vi "neo.vi"() -> ()   [LabVIEW 2012]
uses:
  E:/Kinect/Neobotix/CSInterface/RosBridgeDotNet.dll
  RosBridgeDotNet.dll
panel:
  out "container2":dbl[](graph)
  in  "MelyIP":u16(ring) items=["192.168.0.152", "127.0.0.1"]
  out "Graph":dbl[](graph)
  in  "gear":i32(knob)=12 scale=20.0..5.0
  in  "0seb":bool
  in  "Jobb":dbl(slide) scale=-2.0..2.0
  in  "Bal":dbl(slide) scale=-2.0..2.0 scale format="%0#1_1g"
  out "Joy":picture
  in  "Disconn":bool
  out "IPEredmeny":T1(array[cluster]) {"Status" items=["Success"=0, "DestinationNetworkUnreachable"=11002, "DestinationHostUnreachable"=11003, "DestinationProhibited, DestinationProtocolUnreachable"=11004, "DestinationPortUnreachable"=11005, "NoResources"=11006, "BadOption"=11007, "HardwareError"=11008, "PacketTooBig"=11009, "TimedOut"=11010, "BadRoute"=11012, "TtlExpired"=11013, "TtlReassemblyTimeExceeded"=11014, "ParameterProblem"=11015, "SourceQuench"=11016, "BadDestination"=11018, "DestinationUnreachable"=11040, "TimeExceeded"=11041, "BadHeader"=11042, "UnrecognizedNextHeader"=11043, "IcmpError"=11044, "DestinationScopeMismatch"=11045, "Unknown"=-1]}
  in  "Ping":bool
  in  "MessN":bool
  out "Error Out":errorcluster
  in  "Connnect":bool
  out "Connected":bool
  in  "Stop Button":bool
  out "container1":dbl[](graph)
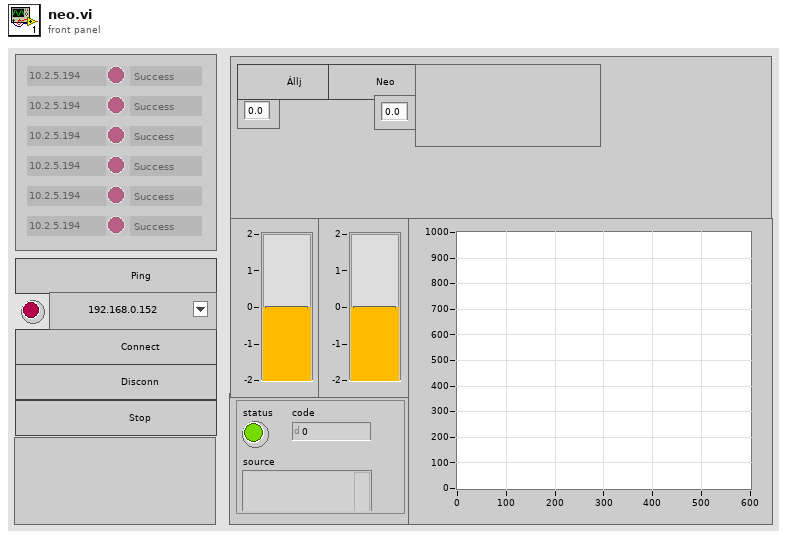
[diagram p1: front panel]
types:
  T1 = cluster{"pingelhet":bool, "IpAddress":string, "Status":i32}[]
  T2 = cluster{"Width":u16, "Style":enum32{"Solid", "Dash", "Dot", "DashDot", "DashDotDot"}}
  T3 = cluster{"left":i16, "top":i16, "right":i16, "bottom":i16}
  T4 = cluster{"pingelhet":bool, "IpAddress":string, "Status":i32}
  T5 = typedef "LVMouseTypeDef.ctl" = cluster{"Mouse Position":cluster{"X":i32, "Y":i32}, "Mouse Modifiers":cluster{"Button Down":bool, "Shift Mod":bool, "Menu Mod":bool, "Option Mod":bool}}
  T6 = typedef "LVBoundsTypeDef.ctl" = cluster{"Width":u32, "Height":u32}
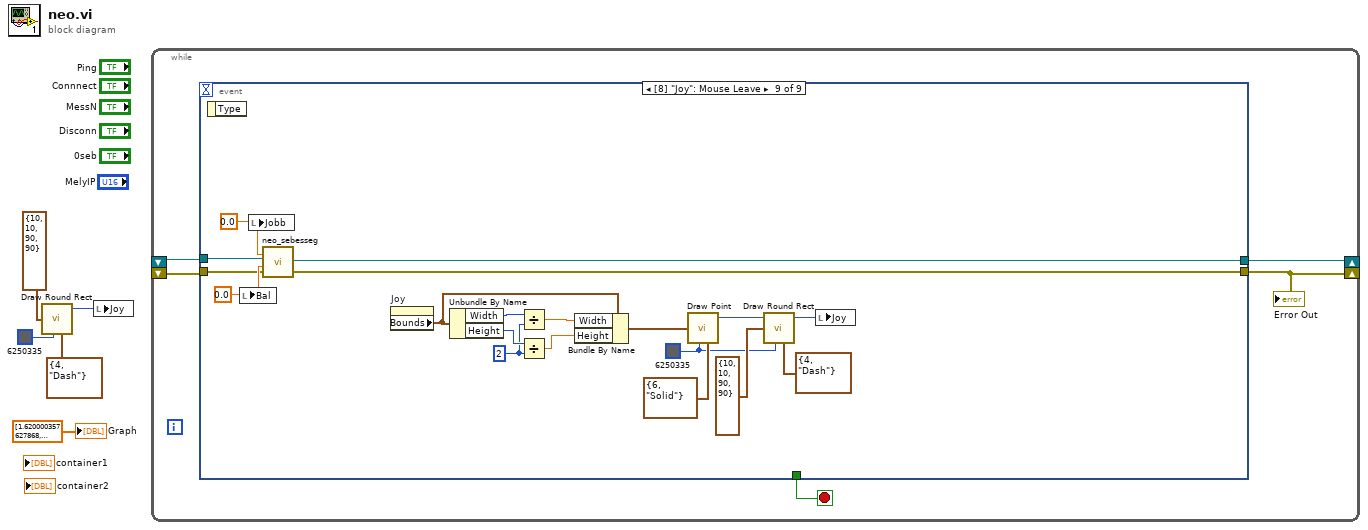
[diagram p0: block diagram]
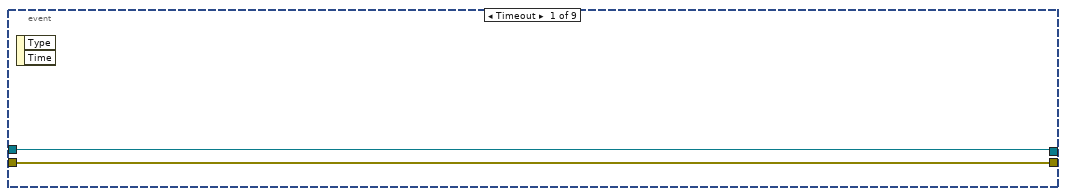
[diagram p2: hidden frame]
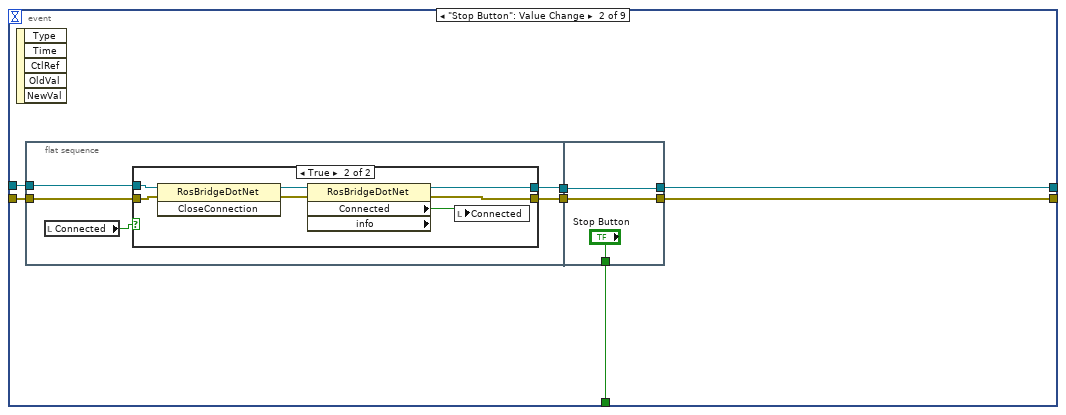
[diagram p3: hidden frame]
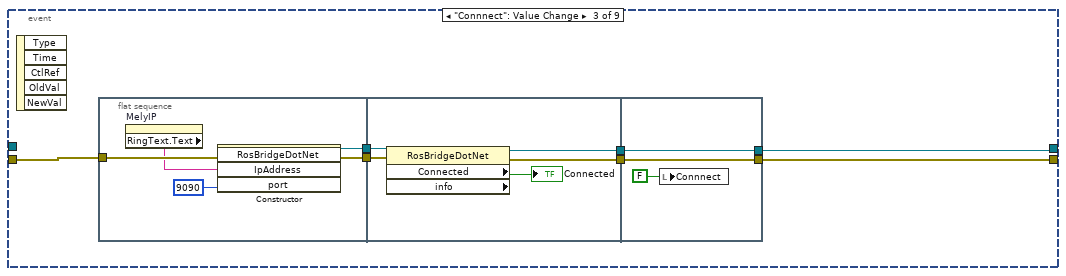
[diagram p5: hidden frame]
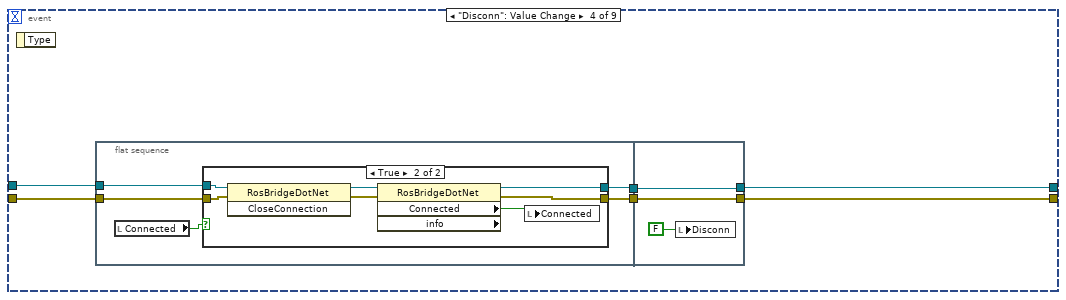
[diagram p6: hidden frame]
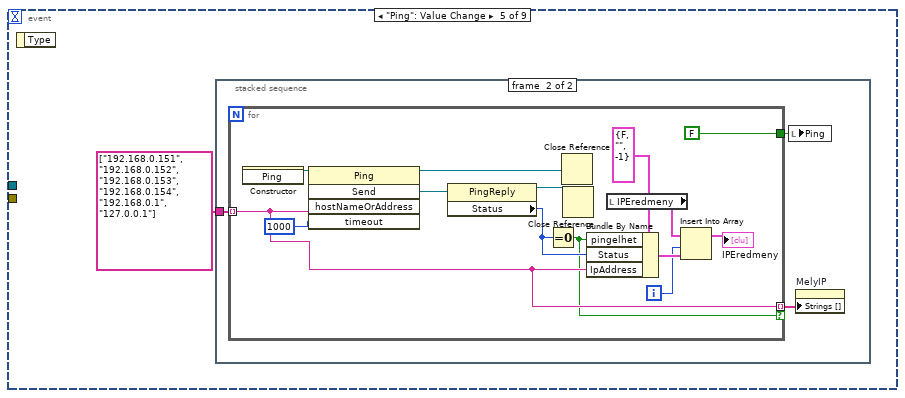
[diagram p8: hidden frame]
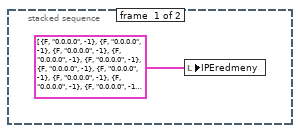
[diagram p9: hidden frame]
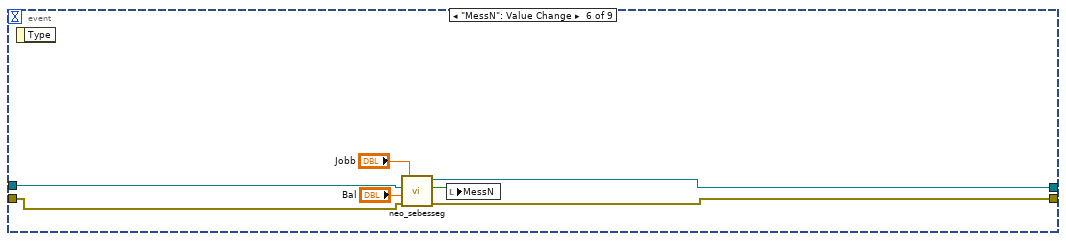
[diagram p10: hidden frame]
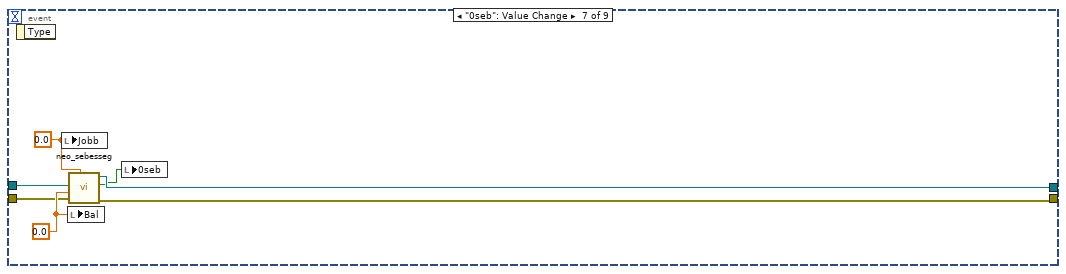
[diagram p11: hidden frame]
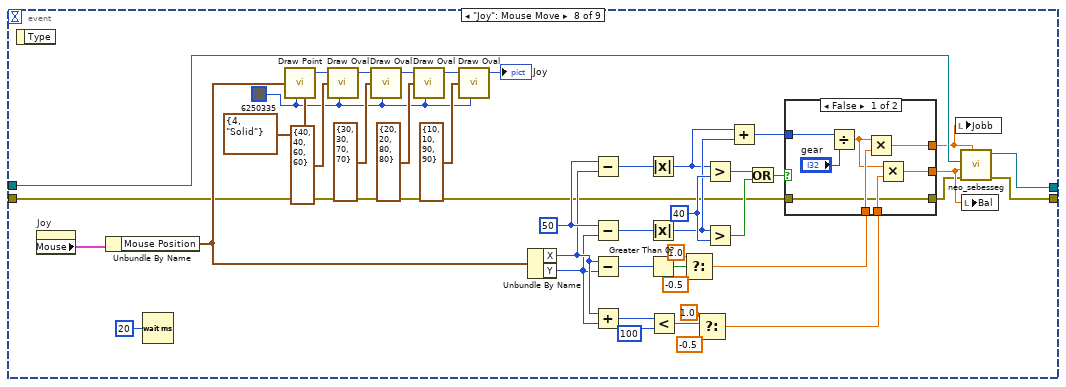
[diagram p12: hidden frame]
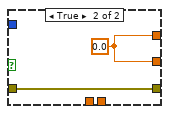
[diagram p13: hidden frame]
diagram:
  n1 = call <vilib>:"Draw Round Rect.vi"("rect"=T3 {"left"=10, "top"=10, "right"=90, "bottom"=90}, "color(black)"=u32 6250335, "pen"=T2 {"Width"=4, "Style"=enum."Dash"}) -> ("new picture"=w1:picture)  [unwired: 6 in]
  n2 = local write "Joy"(w1) -> ()
  n3 = while {
    shift-right: [w9] -> _
    shift-left: _ -> [w7]
    shift-right: [w6] -> _
    shift-left: _ -> [w8]
    stop <- w10 stop-if-true
    n4 = event shown="[8] \"Joy\": Mouse Leave" {
      selector: _ -> [_ _ _ _ _ _ _ _ _]
      dyn-events: _ -> [_ _ _ _ _ _ _ _ _]
      timeout: _ -> [_ _ _ _ _ _ _ _ _]
      tunnel: [_ w13 _ _ _ _ _ _ _] -> w10
      tunnel: [w12 w17 w37 w58 _ w103 w111 w146 w180] -> w9
      tunnel: [w11 w16 w38 w57 _ w102 w107 w147 w181] -> w6
      tunnel: w8 -> [w11 w18 w43 w59 _ w104 w108 w114 w182]
      tunnel: w7 -> [w12 w19 _ w60 _ w105 w112 w148 w183]
      event Timeout {
        n5 = event-data() -> ()  [unwired: 1 in, 2 out]
      }
      event "Stop Button": Value Change {
        n6 = event-data() -> ()  [unwired: 1 in, 5 out]
        n7 = flat-sequence {
          tunnel: w19 -> [w24]
          tunnel: w18 -> [w23]
          tunnel: [w22] -> w15
          tunnel: [w21] -> w14
          tunnel: [w35] -> w16
          tunnel: [w36] -> w17
          tunnel: w15 -> [w36]
          tunnel: w14 -> [w35]
          tunnel: ["Stop Button"] -> w13
          frame #0 {
            n8 = local read "Connected"() -> (w20:bool)
            n9 = case shown="True" w20 {
              tunnel: w24 -> [w26 w31]
              tunnel: w23 -> [w25 w30]
              tunnel: [w26 w29] -> w22
              tunnel: [w25 w28] -> w21
              frame False {
              }
              frame True {
                n10 = invoke class="RosBridgeDotNet" method="CloseConnection"(reference=w31, error in=w30) -> (reference out=w32:refnum<k24>, error out=w33:errorcluster)  [unwired: 1 in, 1 out]
                n11 = property class="RosBridgeDotNet" props=["Connected", "info"](reference=w32, error in=w33) -> (reference out=w29:refnum<k24>, error out=w28:errorcluster, "Connected"=w27:bool)  [unwired: 1 out]
                n12 = local write "Connected"(w27) -> ()
              }
            }
          }
          frame #1 {
          }
        }
      }
      event "Connnect": Value Change {
        n13 = event-data() -> ()  [unwired: 1 in, 5 out]
        n14 = flat-sequence {
          tunnel: [w47] -> w42
          tunnel: [w46] -> w41
          tunnel: w43 -> [w45]
          tunnel: w42 -> [w52]
          tunnel: w41 -> [w51]
          tunnel: [w50] -> w40
          tunnel: [w49] -> w39
          tunnel: w40 -> [w54]
          tunnel: w39 -> [w55]
          tunnel: [w55] -> w38
          tunnel: [w54] -> w37
          frame #0 {
            n15 = property on="MelyIP" class="Ring (strict)"() -> ("RingText.Text"=w44:string)  [unwired: 2 in, 2 out]
            n16 = constructor class="RosBridgeDotNet"(error in=w45, "IpAddress"=w44, "port"=9090) -> (reference out=w47:refnum<k24>, error out=w46:errorcluster)  [unwired: 2 in, 3 out]
          }
          frame #1 {
            n17 = property class="RosBridgeDotNet" props=["Connected", "info"](reference=w52, error in=w51) -> (reference out=w50:refnum<k24>, error out=w49:errorcluster, "Connected"=→"Connected":bool)  [unwired: 1 out]
          }
          frame #2 {
            n18 = local write "Connnect"(FALSE ("Connnect")) -> ()
          }
        }
      }
      event "Disconn": Value Change {
        n19 = event-data() -> ()  [unwired: 1 in, 1 out]
        n20 = flat-sequence {
          tunnel: w60 -> [w67]
          tunnel: w59 -> [w66]
          tunnel: [w65] -> w62
          tunnel: [w64] -> w61
          tunnel: [w78] -> w57
          tunnel: [w79] -> w58
          tunnel: w62 -> [w79]
          tunnel: w61 -> [w78]
          frame #0 {
            n21 = local read "Connected"() -> (w63:bool)
            n22 = case shown="True" w63 {
              tunnel: w67 -> [w69 w74]
              tunnel: w66 -> [w68 w73]
              tunnel: [w69 w72] -> w65
              tunnel: [w68 w71] -> w64
              frame False {
              }
              frame True {
                n23 = invoke class="RosBridgeDotNet" method="CloseConnection"(reference=w74, error in=w73) -> (reference out=w75:refnum<k24>, error out=w76:errorcluster)  [unwired: 1 in, 1 out]
                n24 = property class="RosBridgeDotNet" props=["Connected", "info"](reference=w75, error in=w76) -> (reference out=w72:refnum<k24>, error out=w71:errorcluster, "Connected"=w70:bool)  [unwired: 1 out]
                n25 = local write "Connected"(w70) -> ()
              }
            }
          }
          frame #1 {
            n26 = local write "Disconn"(FALSE ("Disconn")) -> ()
          }
        }
      }
      event "Ping": Value Change {
        n27 = event-data() -> ()  [unwired: 1 in, 1 out]
        n28 = stacked-sequence {
          tunnel: string[] ["192.168.0.151", "192.168.0.152", "192.168.0.153", "192.168.0.154", "192.168.0.1", "127.0.0.1"] ("IPCimek 3") -> [_ w83]
          frame #0 {
            n29 = local write "IPEredmeny"(T1 [{"pingelhet"=FALSE, "IpAddress"="0.0.0.0", "Status"=-1}, {"pingelhet"=FALSE, "IpAddress"="0.0.0.0", "Status"=-1}, {"pingelhet"=FALSE, "IpAddress"="0.0.0.0", "Status"=-1}, {"pingelhet"=FALSE, "IpAddress"="0.0.0.0", "Status"=-1}, {"pingelhet"=FALSE, "IpAddress"="0.0.0.0", "Status"=-1}, {"pingelhet"=FALSE, "IpAddress"="0.0.0.0", "Status"=-1}, {"pingelhet"=FALSE, "IpAddress"="0.0.0.0", "Status"=-1}, {"pingelhet"=FALSE, "IpAddress"="0.0.0.0", "Status"=-1}, {"pingelhet"=FALSE, "IpAddress"="0.0.0.0", "Status"=-1}, {"pingelhet"=FALSE, "IpAddress"="0.0.0.0", "Status"=-1}, {"pingelhet"=FALSE, "IpAddress"="0.0.0.0", "Status"=-1}] ("IPEredmeny 2")) -> ()
          }
          frame #1 {
            n30 = for {
              tunnel: [FALSE ("Ping")] -> w84
              tunnel: w83 -> [w86] mode=indexing
              tunnel: [w86] -> w82 mode=indexing if=w85
              i -> [w90]
              n31 = constructor class="Ping"() -> (reference out=w97:refnum<k24>)  [unwired: 3 in, 2 out]
              n32 = invoke class="Ping" method="Send"(reference=w97, "hostNameOrAddress"=w86, "timeout"=1000) -> (reference out=w95:refnum<k24>, "Send"=w98:refnum<k24>)  [unwired: 2 in, 3 out]
              n33 = property class="PingReply"(reference=w98) -> (reference out=w96:refnum<k24>, "Status"=w93:i32)  [unwired: 1 in, 1 out]
              n34 = Equal To 0?(x=w93) -> (x = 0?=w85:bool)
              n35 = Close Reference(reference=w95) -> ()  [unwired: 1 in, 1 out]
              n36 = Close Reference(reference=w96) -> ()  [unwired: 1 in, 1 out]
              n37 = Bundle By Name(cluster=T4 {"pingelhet"=FALSE, "IpAddress"="", "Status"=-1} ("element"), "pingelhet"=w85, "Status"=w93, "IpAddress"=w86) -> (w91:T4)
              n38 = local read "IPEredmeny"() -> (w87:T1)
              n39 = Insert Into Array(array=w87, index=w90, new element=w91) -> (→"IPEredmeny":T1)
            }
            n40 = local write "Ping"(w84) -> ()
            n41 = property on="MelyIP" class="Ring (strict)"("Strings []"=w82) -> ()  [unwired: 2 in, 2 out]
          }
        }
      }
      event "MessN": Value Change {
        n42 = event-data() -> ()  [unwired: 1 in, 1 out]
        n43 = call "neo_sebesseg.vi"("Jobb"="Jobb", "error in (no error)"=w104, "Bal"="Bal", "new reference in"=w105) -> ("error out"=w102:errorcluster, "vissza"=w99:bool, ".NET Refnum out"=w103:refnum<k24>)  [unwired: 5 in]
        n44 = local write "MessN"(w99) -> ()
      }
      event "0seb": Value Change {
        w110 = 0.0 ("element")
        w109 = 0.0 ("element")
        n45 = event-data() -> ()  [unwired: 1 in, 1 out]
        n46 = local write "Jobb"(w110) -> ()
        n47 = local write "Bal"(w109) -> ()
        n48 = call "neo_sebesseg.vi"("Jobb"=w110, "error in (no error)"=w108, "Bal"=w109, "new reference in"=w112) -> ("error out"=w107:errorcluster, "vissza"=w106:bool, ".NET Refnum out"=w111:refnum<k24>)  [unwired: 5 in]
        n49 = local write "0seb"(w106) -> ()
      }
      event "Joy": Mouse Move {
        w115 = u32 6250335
        w139 = 40 ("y")
        w140 = 50
        n50 = event-data() -> ()  [unwired: 1 in, 1 out]
        n51 = property on="Joy" class="Pict"() -> ("Mouse"=w156:T5)  [unwired: 2 in, 2 out]
        n52 = Unbundle By Name(w156) -> ("Mouse Position"=w142:cluster{"X":i32, "Y":i32})
        n53 = Wait (ms)(milliseconds to wait=u32 20) -> ()  [unwired: 1 out]
        n54 = call <vilib>:"Draw Point.vi"("point(x,y)"=w142, "color(black)"=w115, "pen"=T2 {"Width"=4, "Style"=enum."Solid"}) -> ("new picture"=w152:picture)  [unwired: 6 in]
        n55 = call <vilib>:"Draw Oval.vi"("picture"=w152, "rect"=T3 {"left"=40, "top"=40, "right"=60, "bottom"=60}, "color(black)"=w115) -> ("new picture"=w154:picture)  [unwired: 6 in]
        n56 = call <vilib>:"Draw Oval.vi"("picture"=w154, "rect"=T3 {"left"=30, "top"=30, "right"=70, "bottom"=70}, "color(black)"=w115) -> ("new picture"=w150:picture)  [unwired: 6 in]
        n57 = call <vilib>:"Draw Oval.vi"("picture"=w150, "rect"=T3 {"left"=20, "top"=20, "right"=80, "bottom"=80}, "color(black)"=w115) -> ("new picture"=w144:picture)  [unwired: 6 in]
        n58 = call <vilib>:"Draw Oval.vi"("picture"=w144, "rect"=T3 {"left"=10, "top"=10, "right"=90, "bottom"=90}, "color(black)"=w115) -> ("new picture"=→"Joy":picture)  [unwired: 6 in]
        n59 = Unbundle By Name(w142) -> ("X"=w133:i32, "Y"=w132:i32)
        n60 = Subtract(x=w140, y=w133) -> (x-y=w129:i32)
        n61 = Subtract(x=w140, y=w132) -> (x-y=w128:i32)
        n62 = Subtract(x=w133, y=w132) -> (x-y=w134:i32)
        n63 = Add(x=w133, y=w132) -> (x+y=w131:i32)
        n64 = Absolute Value(x=w129) -> (abs(x)=w118:i32)
        n65 = Absolute Value(x=w128) -> (abs(x)=w119:i32)
        n66 = Greater Than 0?(x=w134) -> (x > 0?=w127:bool)
        n67 = Less?(x=w131, y=100) -> (x < y?=w122:bool)
        n68 = Select(t=1.0, s=w127, f=-0.5) -> (s? t:f=w124:dbl)
        n69 = Select(t=1.0, s=w122, f=-0.5) -> (s? t:f=w120:dbl)
        n70 = Greater?(x=w118, y=w139) -> (0:w137:bool)
        n71 = Greater?(x=w119, y=w139) -> (0:w138:bool)
        n72 = Add(x=w118, y=w119) -> (x+y=w117:i32)
        n73 = Or(x=w137, y=w138) -> (x .or. y?=w141:bool)
        n74 = case shown="False" w141 {
          tunnel: [w163 w166] -> w135
          tunnel: [w160 w166] -> w136
          tunnel: w117 -> [w164 _]
          tunnel: w124 -> [w162 _]
          tunnel: w120 -> [w161 _]
          tunnel: w114 -> [w157 w165]
          tunnel: [w157 w165] -> w113
          frame False {
            n75 = Divide(x=w164, y="gear") -> (x/y=w159:dbl)
            n76 = Multiply(x=w159, y=w162) -> (x*y=w163:dbl)
            n77 = Multiply(x=w159, y=w161) -> (x*y=w160:dbl)
          }
          frame True {
            w166 = 0.0 ("Jobb")
          }
        }
        n78 = local write "Jobb"(w135) -> ()
        n79 = call "neo_sebesseg.vi"("Jobb"=w135, "error in (no error)"=w113, "Bal"=w136, "new reference in"=w148) -> ("error out"=w147:errorcluster, ".NET Refnum out"=w146:refnum<k24>)  [unwired: 5 in, 1 out]
        n80 = local write "Bal"(w136) -> ()
      }
      event "Joy": Mouse Leave {
        w167 = u32 6250335
        w177 = u32 2 ("y")
        w185 = 0.0 ("element")
        w184 = 0.0 ("element")
        n81 = event-data() -> ()  [unwired: 1 in, 1 out]
        n82 = local write "Bal"(w184) -> ()
        n83 = local write "Jobb"(w185) -> ()
        n84 = call "neo_sebesseg.vi"("Jobb"=w185, "error in (no error)"=w182, "Bal"=w184, "new reference in"=w183) -> ("error out"=w181:errorcluster, ".NET Refnum out"=w180:refnum<k24>)  [unwired: 5 in, 1 out]
        n85 = property on="Joy" class="Pict"() -> ("Bounds"=w175:T6)  [unwired: 2 in, 2 out]
        n86 = Unbundle By Name(w175) -> ("Width"=w179:u32, "Height"=w178:u32)
        n87 = Divide(x=w179, y=w177) -> (x/y=w176:dbl)
        n88 = Divide(x=w178, y=w177) -> (x/y=w174:dbl)
        n89 = Bundle By Name(cluster=w175, "Width"=w176, "Height"=w174) -> (w172:T6)
        n90 = call <vilib>:"Draw Point.vi"("point(x,y)"=w172, "color(black)"=w167, "pen"=T2 {"Width"=6, "Style"=enum."Solid"}) -> ("new picture"=w171:picture)  [unwired: 6 in]
        n91 = call <vilib>:"Draw Round Rect.vi"("picture"=w171, "rect"=T3 {"left"=10, "top"=10, "right"=90, "bottom"=90}, "color(black)"=w167, "pen"=T2 {"Width"=4, "Style"=enum."Dash"}) -> ("new picture"=w170:picture)  [unwired: 5 in]
        n92 = local write "Joy"(w170) -> ()
      }
    }
    "Error Out" <- w6
  }
  "Graph" <- dbl[] [1.620000357627868, 14.61999988079071, 23.620000238418577, 28.620001430511476, 31.619998569488526, 31.619998569488526, 33.619999642372136, 34.61999868869782, 34.61999868869782, 36.619999761581425, 39.619999880790715, 37.61999880790711, 39.619999880790715, 39.619999880790715, 40.6199989271164, 42.620000000000005, 43.61999904632569, 45.619997138977055, 45.619997138977055, 48.620000238418584, 48.620000238418584, 49.61999928474427, 48.620000238418584, 49.61999928474427, 49.61999928474427, 49.61999928474427, 50.61999833106995, 49.61999928474427, 48.620000238418584, 48.620000238418584, 50.61999833106995, 48.620000238418584, 48.620000238418584, 48.620000238418584, 48.620000238418584, 47.6200011920929, 48.620000238418584, 48.620000238418584, 45.619997138977055, 41.62000095367432, 34.61999868869782, 30.619999523162843, 31.619998569488526, 24.61999928474426, 18.61999904632568, 12.620000298023223, 24.61999928474426, 29.62000047683716, 41.62000095367432, -1.380000134110451, 216.62000095367432, 198.61999427795408, 189.62000286102293, 189.62000286102293, 179.62000047683713, 207.62000953674317, 203.61998950958252, 188.62000381469724, 189.62000286102293, 204.6199885559082, 267.62, 287.6200047683716, 288.62000381469727, 289.62000286102295, 621.6199961853027, 612.6199809265137, 610.6199828338623, 625.6199923706055, 629.6199885559082, 626.6200152587891, 624.6200171661377, 612.6199809265137, 627.6199904632568, 640.6200019073486, 626.6200152587891, 567.62, 562.6199809265137, 558.6199847412109, 559.6200076293945, 557.6200095367432, 558.6199847412109, 557.6200095367432, 556.6199866485596, 553.6200133514404, 551.6200152587891, 557.6200095367432, 561.6200057220459, 561.6200057220459, 561.6200057220459, 563.6200038146973, 539.619979019165, 458.6199847412109, 441.61997711181635, 451.620015258789, 560.6199828338623, 266.6200009536743, 265.62000190734864, 265.62000190734864, 267.62, 561.6200057220459, 562.6199809265137, 563.6200038146973, 564.619979019165, 576.6200152587891, 636.6200057220459, 637.6199809265137, 639.619979019165, 640.6200019073486, 639.619979019165, 442.61999999999995, 443.62002288818354, 645.620020980835, 452.6199904632568, 442.61999999999995, 276.61999141693116, 275.6199923706055, 275.6199923706055, 297.6199952316284, 334.62000762939454, 331.6200104904175, 329.6199885559082, 325.6199923706055, 324.6199933242798, 322.6199952316284, 322.6199952316284, 321.61999618530274, 319.6199980926514, 318.6199990463257, 291.6200009536743, 293.6199990463257, 293.6199990463257, 294.6199980926514, 296.61999618530274, 319.6199980926514, 318.6199990463257, 318.6199990463257, 299.6199933242798, 301.61999141693116, 303.6199895095825, 304.6199885559082, 306.6200104904175, 308.62000858306885, 323.6199942779541, 325.6199923706055, 326.61999141693116, 315.62000190734864, 290.62000190734864, 287.6200047683716, 476.620015258789, 478.6200133514404, 474.62001716613764, 457.6200095367431, 458.6199847412109, 477.6199904632568, 541.6199771118164, 259.62000762939454, 256.6200104904175, 253.61998950958252, 254.6199885559082, 251.61999141693116, 259.62000762939454, 317.62, 329.6199885559082, 335.6200066757202, 335.6200066757202, 580.6200114440918, 2988.6199084472655, 340.62000190734864, 342.62, 296.61999618530274, 291.6200009536743, 287.6200047683716, 287.6200047683716, 284.62000762939454, 282.62000953674317, 283.62000858306885, 303.6199895095825, 346.61999618530274, 427.6199904632568, 432.6200095367431, 447.6200190734863, 443.62002288818354, 435.61998283386225, 455.62001144409174, 457.6200095367431, 482.6200095367431, 382.62000953674317, 356.6200104904175, 313.62000381469727, 376.61999141693116, 469.6199980926513, 464.619979019165, 454.61998855590815, 457.6200095367431, 443.62002288818354, 452.6199904632568, 370.61999713897706, 350.6199923706055, 370.61999713897706, 360.6200066757202, 442.61999999999995, 432.6200095367431, 434.6200076293945, 434.6200076293945, 432.6200095367431, 402.6199904632568, 390.62000190734864, 386.6200057220459, 386.6200057220459, 384.62000762939454, 382.62000953674317, 381.6200104904175, 379.6199885559082, 377.61999046325684, 377.61999046325684, 382.62000953674317, 388.62000381469727, 380.6200114440918, 354.6199885559082, 355.6200114440918, 341.6200009536743, 337.6200047683716, 93.61999904632569, 94.61999809265137, 93.61999904632569, 91.62000095367432, 91.62000095367432, 91.62000095367432, 90.62000190734864, 91.62000095367432, 89.62000286102295, 89.62000286102295, 90.62000190734864, 91.62000095367432, 91.62000095367432, 89.62000286102295, 89.62000286102295, 89.62000286102295, 89.62000286102295, 89.62000286102295, 90.62000190734864, 89.62000286102295, 88.61999785423279, 88.61999785423279, 86.61999976158143, 88.61999785423279, 88.61999785423279, 87.61999880790711, 88.61999785423279, 88.61999785423279, 89.62000286102295, 88.61999785423279, 87.61999880790711, 89.62000286102295, 88.61999785423279, 88.61999785423279, 87.61999880790711, 87.61999880790711, 88.61999785423279, 87.61999880790711, 88.61999785423279, 87.61999880790711, 87.61999880790711, 87.61999880790711, 88.61999785423279, 88.61999785423279, 88.61999785423279, 87.61999880790711, 87.61999880790711, 88.61999785423279, 88.61999785423279, 86.61999976158143, 88.61999785423279, 88.61999785423279, 88.61999785423279, 88.61999785423279, 88.61999785423279, 88.61999785423279, 87.61999880790711, 88.61999785423279, 88.61999785423279, 88.61999785423279, 88.61999785423279, 89.62000286102295, 88.61999785423279, 90.62000190734864, 89.62000286102295, 89.62000286102295, 90.62000190734864, 90.62000190734864, 90.62000190734864, 90.62000190734864, 90.62000190734864, 90.62000190734864, 90.62000190734864, 90.62000190734864, 92.62, 93.61999904632569, 324.6199933242798, 324.6199933242798, 326.61999141693116, 326.61999141693116, 328.6199895095825, 329.6199885559082, 329.6199885559082, 331.6200104904175, 332.62000953674317, 332.62000953674317, 334.62000762939454, 336.6200057220459, 337.6200047683716, 339.62000286102295, 339.62000286102295, 341.6200009536743, 342.62, 343.6199990463257, 345.61999713897706, 346.61999618530274, 347.6199952316284, 228.61998950958252, 211.6200057220459, 206.62001049041749, 202.61999046325684, 199.61999332427976, 196.6199961853027, 193.61999904632566, 190.6200019073486, 187.62000476837156, 185.61999475479124, 186.62000572204587, 185.61999475479124, 188.62000381469724, 189.62000286102293, 190.6200019073486, 191.6200009536743, 193.61999904632566, 193.61999904632566, 195.61999713897703, 196.6199961853027, 197.6199952316284, 199.61999332427976, 201.61999141693116, 202.61999046325684, 204.6199885559082, 371.61999618530274, 371.61999618530274, 372.6199952316284, 379.6199885559082, 2988.6199084472655, 435.61998283386225, 440.6200019073486, 443.62002288818354, 446.6199961853027, 451.620015258789, 453.6200133514404, 459.6200076293945, 462.6199809265136, 467.61999999999995, 471.6199961853027, 476.620015258789, 480.62001144409174, 484.6200076293945, 489.619979019165, 489.619979019165, 486.62000572204585, 491.61997711181635, 496.6199961853027, 498.61999427795405, 503.6200133514404, 510.61998283386225, 515.6200019073486, 521.6199961853027, 528.6200133514404, 534.6200076293945, 542.62, 548.6199942779541, 555.6200114440918, 561.6200057220459, 350.6199923706055, 349.6199933242798, 349.6199933242798, 175.6200042915344, 175.6200042915344, 177.62000238418577, 189.62000286102293, 335.6200066757202, 169.61999809265134, 167.61999999999998, 165.6200019073486, 166.6200009536743, 164.62000286102293, 163.62000381469724, 163.62000381469724, 157.61999761581419, 151.62000333786008, 151.62000333786008, 158.61999666213987, 161.62000572204587, 165.6200019073486, 167.61999999999998, 169.61999809265134, 172.6199952316284, 176.62000333786008, 179.62000047683713, 192.61999999999998, 210.62000667572022, 473.61999427795405, 673.6199942779541, 672.6200190734863, 206.62001049041749, 211.6200057220459, 172.6199952316284, 183.61999666213987, 212.6200047683716, 211.6200057220459, 229.6199885559082, 229.6199885559082, 229.6199885559082, 230.6200114440918, 229.6199885559082, 238.62000381469727, 365.62000190734864, 528.6200133514404, 2988.6199084472655, 376.61999141693116, 52.620002384185796, 50.61999833106995, 50.61999833106995, 50.61999833106995, 50.61999833106995, 49.61999928474427, 48.620000238418584, 47.6200011920929, 48.620000238418584, 47.6200011920929, 48.620000238418584, 48.620000238418584, 48.620000238418584, 48.620000238418584, 49.61999928474427, 50.61999833106995, 51.619997377395634, 53.62000143051148, 52.620002384185796, 55.619999523162846, 57.61999761581421, 57.61999761581421, 58.620002622604375, 66.62000095367432, 834.6200076293945, 834.6200076293945, 57.61999761581421, 56.61999856948853, 53.62000143051148, 53.62000143051148, 53.62000143051148, 51.619997377395634, 51.619997377395634, 50.61999833106995, 49.61999928474427, 48.620000238418584, 48.620000238418584, 48.620000238418584, 47.6200011920929, 47.6200011920929, 46.62000214576722, 47.6200011920929, 45.619997138977055, 46.62000214576722, 46.62000214576722, 46.62000214576722, 44.61999809265137, 45.619997138977055, 45.619997138977055, 45.619997138977055, 45.619997138977055, 45.619997138977055, 45.619997138977055, 46.62000214576722, 46.62000214576722, 47.6200011920929, 47.6200011920929, 48.620000238418584, 48.620000238418584, 48.620000238418584, 48.620000238418584, 369.6199980926514, 362.6200047683716, 1.620000357627868, 1.620000357627868, 2.6200001490116116, 5.619999523162841, 8.61999964237213, 17.619999999999997, 22.620001192092893, 28.620001430511476, 29.62000047683716, 34.61999868869782, 39.619999880790715, 41.62000095367432, 41.62000095367432, 44.61999809265137, 46.62000214576722, 44.61999809265137, 43.61999904632569, 47.6200011920929, 47.6200011920929, 47.6200011920929, 47.6200011920929, 46.62000214576722, 45.619997138977055, 46.62000214576722, 46.62000214576722, 45.619997138977055, 47.6200011920929, 46.62000214576722, 45.619997138977055, 43.61999904632569, 42.620000000000005, 41.62000095367432, 42.620000000000005, 40.6199989271164, 41.62000095367432, 40.6199989271164, 38.62000083446503, 38.62000083446503, 39.619999880790715, 36.619999761581425, 37.61999880790711, 34.61999868869782, 36.619999761581425, 35.62000071525574, 36.619999761581425, 35.62000071525574, 29.62000047683716, 28.620001430511476, 24.61999928474426, 17.619999999999997, -1.380000134110451, -1.380000134110451] ("Array")
